vi "smooth test data.vi"(8 "smooth point":dbl, 9 "input array":dbl[](array[numeric]), 10 "test item name smooth":string[](array[string]), 11 "test item name":string) -> (3 "output array":dbl[](array[numeric]))   [LabVIEW 2011]
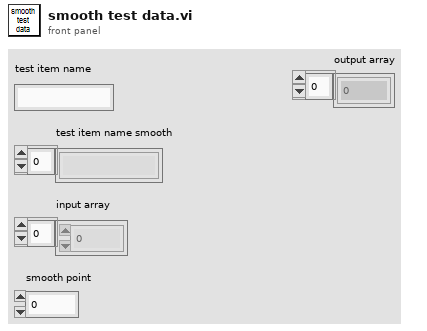
[diagram p1: front panel]
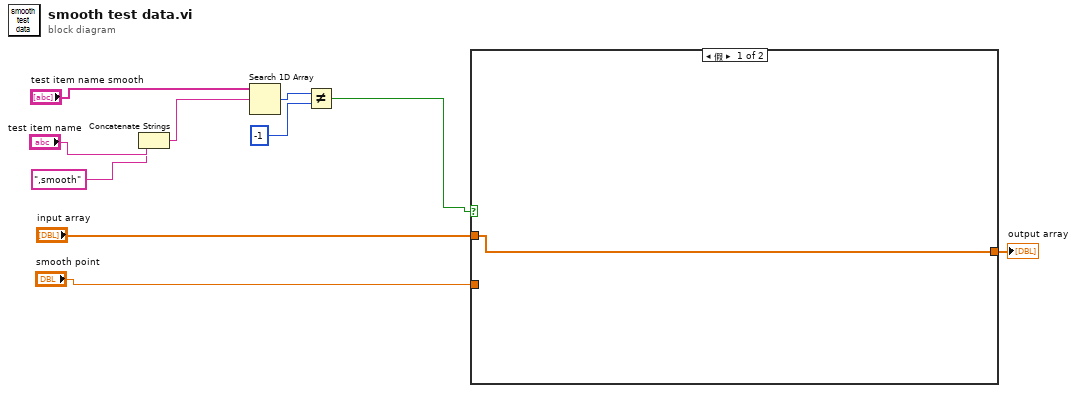
[diagram p0: block diagram]
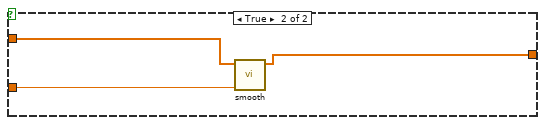
[diagram p2: hidden frame]
diagram:
  n1 = Concatenate Strings("test item name", ",smooth" ("字符串")) -> (w8:string)
  n2 = Search 1D Array(1D array="test item name smooth", element=w8) -> (index of element=w6:i32)  [unwired: 1 in]
  n3 = Not Equal?(x=w6, y=-1) -> (x != y?=w4:bool)
  n4 = case shown="假" w4 {
    tunnel: "input array" -> [w11 w14]
    tunnel: "smooth point" -> [_ w13]
    tunnel: [w11 w12] -> w1
    frame False {
    }
    frame True {
      n5 = call "smooth.vi"("point"=w13, "input array"=w14) -> ("output array"=w12:dbl[])  [unwired: 9 in]
    }
  }
  "output array" <- w1
